vi "LoadSymbolNames.vi"(8 "error in (no error)":errorcluster, 11 "TCatAdsNet in":refnum<class "AdsNET.lvclass">) -> (0 "error out":errorcluster, 2 "SymbolNameList":string[](array[string]), 3 "TCatAdsNet out":refnum<class "AdsNET.lvclass">)   [LabVIEW 2016, in "TCatAdsNet.lvlib" / "AdsNET.lvclass"]
uses:
  AdsNET.lvclass
  AdsNET.lvclass/AdsNET.ctl
  C:/Users/Maurizio/Projects/sentiero-beckoff/DLL/TwinCAT.Ads.dll
  sentiero-beckoff/DLL/TwinCAT.Ads.dll
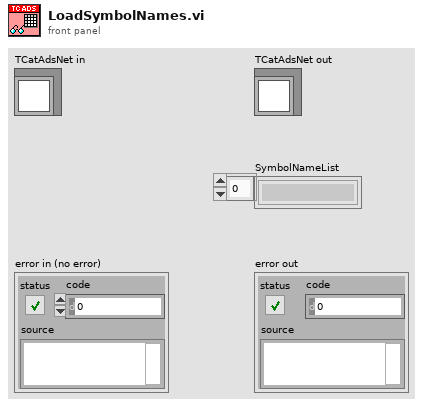
[diagram p1: front panel]
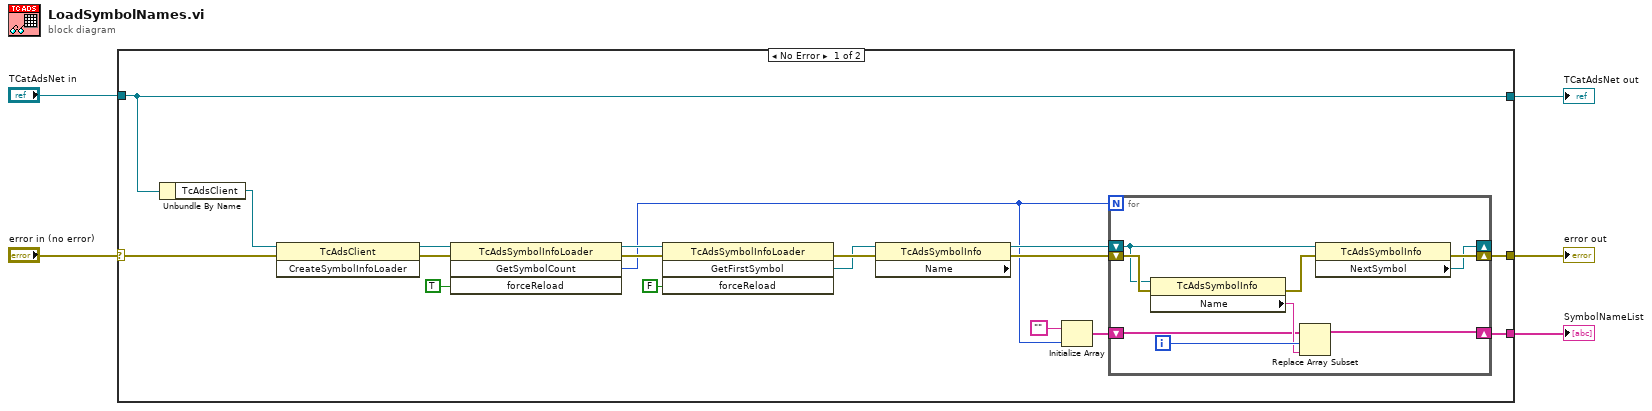
[diagram p0: block diagram]
diagram:
  n1 = case shown="No Error" "error in (no error)" {
    selector: "error in (no error)" -> [w7 w33]
    tunnel: "TCatAdsNet in" -> [w6 w34]
    tunnel: [w6 w34] -> w4
    tunnel: [w10 w33] -> w3
    tunnel: [w9 _] -> w2
    frame No Error {
      n2 = Unbundle By Name(w6) -> ("TcAdsClient"=w23:refnum<k24>)
      n3 = invoke class="TcAdsClient" method="CreateSymbolInfoLoader"(reference=w23, error in=w7) -> (error out=w11:errorcluster, "CreateSymbolInfoLoader"=w12:refnum<k24>)  [unwired: 1 in, 1 out]
      n4 = invoke class="TcAdsSymbolInfoLoader" method="GetSymbolCount"(reference=w12, error in=w11, "forceReload"=TRUE) -> (reference out=w13:refnum<k24>, error out=w15:errorcluster, "GetSymbolCount"=w8:i32)  [unwired: 1 in, 1 out]
      n5 = invoke class="TcAdsSymbolInfoLoader" method="GetFirstSymbol"(reference=w13, error in=w15, "forceReload"=FALSE) -> (error out=w20:errorcluster, "GetFirstSymbol"=w19:refnum<k24>)  [unwired: 1 in, 2 out]
      n6 = property class="TcAdsSymbolInfo" props=["Name"](reference=w19, error in=w20) -> (reference out=w22:refnum<k24>, error out=w21:errorcluster)  [unwired: 1 out]
      n7 = Initialize Array("", w8) -> (w14:string[])
      n8 = for {
        N: w8 -> [_]
        shift-right: [w29] -> w10
        shift-left: w21 -> [w31]
        shift-right: [w26] -> _
        shift-left: w22 -> [w27]
        shift-right: [w24] -> w9
        shift-left: w14 -> [w25]
        i -> [w32]
        n9 = property class="TcAdsSymbolInfo"(reference=w27, error in=w31) -> (error out=w30:errorcluster, "Name"=w28:string)  [unwired: 1 out]
        n10 = Replace Array Subset(array=w25, new element=w28, index=w32) -> (w24:string[])
        n11 = property class="TcAdsSymbolInfo"(reference=w27, error in=w30) -> (error out=w29:errorcluster, "NextSymbol"=w26:refnum<k24>)  [unwired: 1 out]
      }
    }
    frame Error {
    }
  }
  "TCatAdsNet out" <- w4
  "error out" <- w3
  "SymbolNameList" <- w2
